vi "Proceed.vi"(7 "component is ready (Y)":bool=TRUE, 8 "error in (no error)":errorcluster, 10 "ProceedMessage":refnum<class "ProceedMessage.lvclass">, 11 "Cascade in":refnum<class "Cascade.lvclass">) -> (0 "error out":errorcluster, 2 "all observers are ready?":bool, 3 "Cascade out":refnum<class "Cascade.lvclass">)   [LabVIEW 2012, in "Cascade.lvclass"]
doc: "The Proceed method is used to check if your component is ready. Also it checks if the observers are ready. When the observers and the component are ready, it sends the proceed to its observee. If it's the highest observee, it distributes a stop command."
uses:
  Cascade.lvclass
  <vilib>/Distrio/Murmex/ProceedMessage/ProceedMessage.lvclass
  Cascade.lvclass/Cascade.ctl
  <vilib>/Distrio/Murmex/Murmex/Murmex.lvclass
panel:
  # "This method is called when the PROCEED\ntrigger is sent. \n\nOverride this method when your component needs to\nrespond to this trigger. \n\nCall parent for proper implementation"
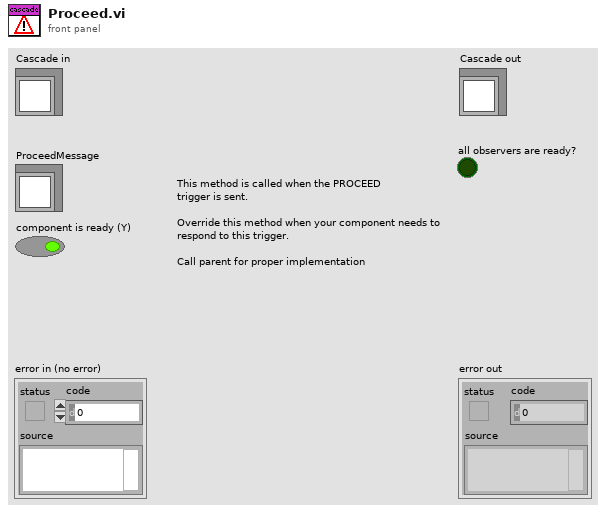
[diagram p1: front panel]
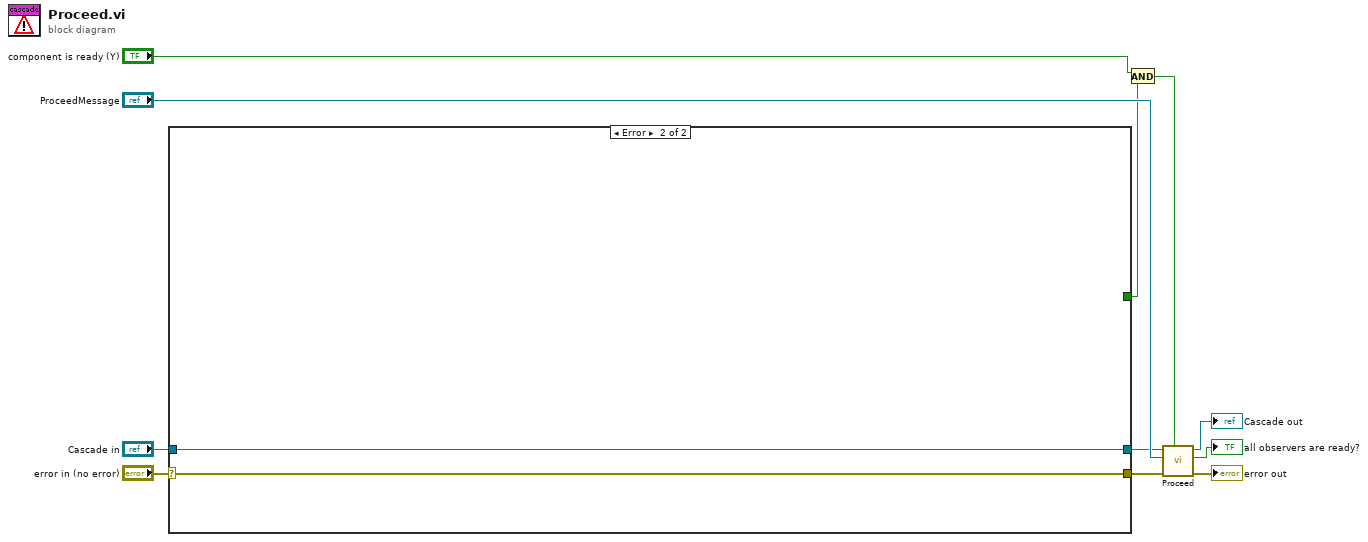
[diagram p0: block diagram]
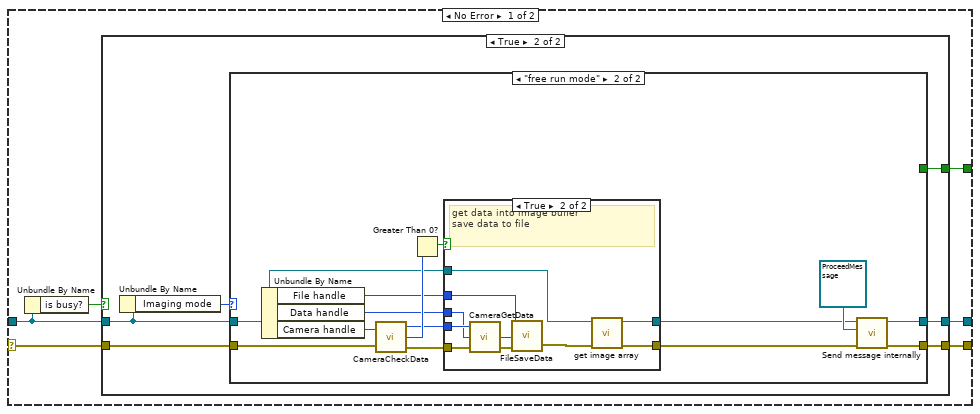
[diagram p2: hidden frame]
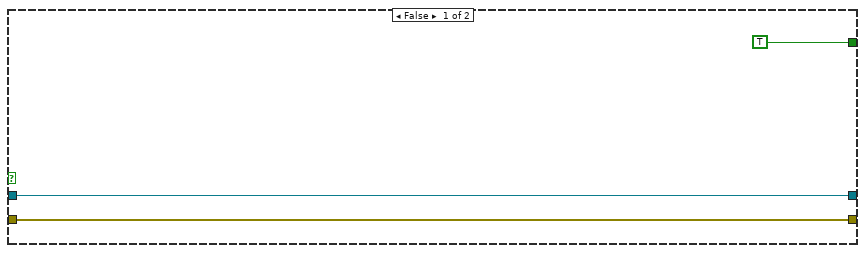
[diagram p3: hidden frame]
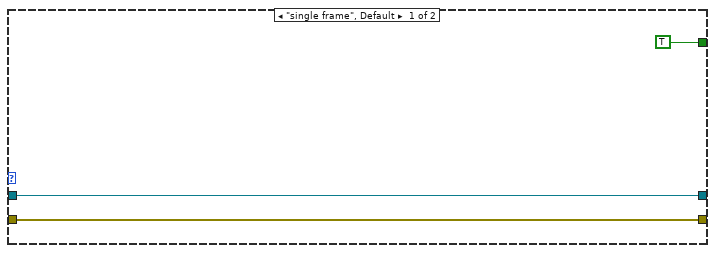
[diagram p4: hidden frame]
diagram:
  n1 = case shown="Error" "error in (no error)" {
    selector: "error in (no error)" -> [w17 w57]
    tunnel: "Cascade in" -> [w16 w56]
    tunnel: [w14 w57] -> w6
    tunnel: [w13 w56] -> w5
    tunnel: [w12 _] -> w3
    frame No Error {
      n2 = Unbundle By Name(w16) -> ("is busy?"=w15:bool)
      n3 = case shown="True" w15 {
        tunnel: w17 -> [w19 w26]
        tunnel: w16 -> [w18 w25]
        tunnel: [w19 w23] -> w14
        tunnel: [w18 w22] -> w13
        tunnel: [TRUE w21] -> w12
        frame False {
        }
        frame True {
          n4 = Unbundle By Name(w25) -> ("Imaging mode"=w24:enum16{"single frame", "free run mode"})
          n5 = case shown="\"free run mode\"" w24 {
            tunnel: w26 -> [w28 w36]
            tunnel: w25 -> [w27 w31]
            tunnel: [w28 w39] -> w23
            tunnel: [w27 w37] -> w22
            tunnel: [TRUE _] -> w21
            frame "single frame", Default {
            }
            frame "free run mode" {
              n6 = Unbundle By Name(w31) -> ("File handle"=w32:u32, "Data handle"=w33:u32, "Camera handle"=w34:u32)
              n7 = call <userlib>:"CameraCheckData.vi"("Camera Handle"=w34, "error in"=w36) -> ("Camera Handle"=w40:u32, "Number Of Frames Available"=w41:i32, "error out"=w43:errorcluster)
              n8 = Greater Than 0?(x=w41) -> (x > 0?=w42:bool)
              n9 = case shown="True" w42 {
                tunnel: w43 -> [w45 w55]
                tunnel: w40 -> [_ w53]
                tunnel: [w45 w48] -> w35
                tunnel: w33 -> [_ w51]
                tunnel: w32 -> [_ w50]
                tunnel: w31 -> [w44 w47]
                tunnel: [w44 w46] -> w30
                frame False {
                }
                frame True {
                  # "get data into image buffer\nsave data to file"
                  n10 = call <userlib>:"CameraGetData.vi"("error in"=w55, "Data Handle"=w51, "Camera Handle"=w53) -> ("error out"=w54:errorcluster, "Data Handle"=w52:u32)  [unwired: 1 out]
                  n11 = call <userlib>:"FileSaveData.vi"("error in"=w54, "Image Handle"=w52, "File Handle"=w50) -> ("error out"=w49:errorcluster)  [unwired: 1 out]
                  n12 = call-dynamic "get image array.vi"("error in (no error)"=w49, "Cascade in"=w47) -> ("error out"=w48:errorcluster, "Cascade out"=w46:refnum<class "Cascade.lvclass">)  [unwired: 8 in]
                }
              }
              n13 = call <vilib>:"Send message internally.vi"("error in (no error)"=w35, "Message"=refnum<class "ProceedMessage.lvclass"> refnum ("Distrio Murmex 1.5:ProceedMessage"), "Murmex in"=w30) -> ("error out"=w39:errorcluster, "Murmex out"=w37:refnum<class "Cascade.lvclass">)  [unwired: 7 in]
            }
          }
        }
      }
    }
    frame Error {
    }
  }
  n14 = And(x="component is ready (Y)", y=w3) -> (x .and. y?=w1:bool)
  n15 = call-parent "Proceed.vi"("component is ready (Y)"=w1, "error in (no error)"=w6, "ProceedMessage"="ProceedMessage", "Murmex in"=w5) -> ("error out"=→"error out":errorcluster, "all observers are ready?"=→"all observers are ready?":bool, "Murmex out"=→"Cascade out":refnum<class "Cascade.lvclass">)  [unwired: 5 in]
